vi "Init.vi"(8 "error in (no error)":errorcluster, 11 "UI in":refnum<class "UI.lvclass">) -> (0 "error out":errorcluster, 3 "UI out":refnum<class "UI.lvclass">)   [LabVIEW 2020, in "UI.lvlib" / "UI.lvclass"]
uses:
  UI.lvclass
  UI.lvclass/UI.ctl
  Read Device.vi
  Read VISA resource name.vi
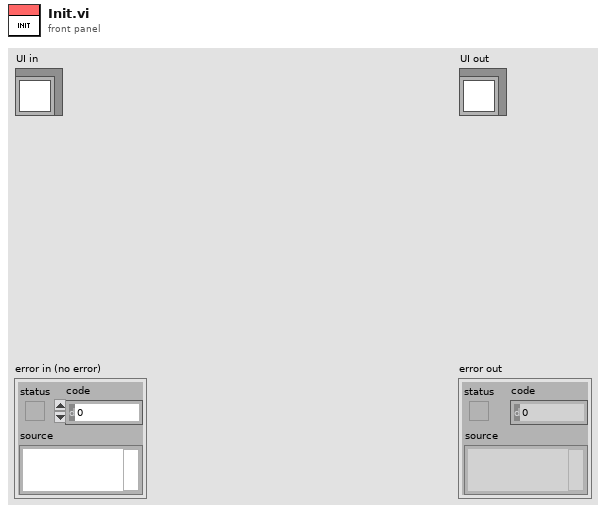
[diagram p1: front panel]
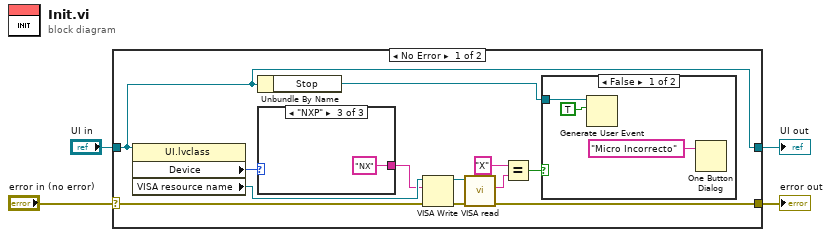
[diagram p0: block diagram]
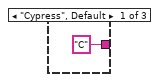
[diagram p3: hidden frame]
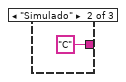
[diagram p4: hidden frame]
diagram:
  n1 = case shown="No Error" "error in (no error)" {
    selector: "error in (no error)" -> [w14 w24]
    tunnel: [w11 w24] -> w3
    tunnel: [w7 w23] -> w1
    tunnel: "UI in" -> [w7 w23]
    frame No Error {
      n2 = property class="UI.lvclass"(reference=w7) -> ("Device"=w16:enum16{"Cypress", "Simulado", "NXP"}, "VISA resource name"=w15:refnum<visa-resource-name>)  [unwired: 1 in, 2 out]
      n3 = Unbundle By Name(w7) -> ("Stop"=w6:refnum<user-event>)
      n4 = case shown="\"NXP\"" w16 {
        tunnel: ["C" "C" "NX"] -> w9
        frame "Cypress", Default {
        }
        frame "Simulado" {
        }
        frame "NXP" {
        }
      }
      n5 = VISA Write(VISA resource name=w15, write buffer=w9, error in (no error)=w14) -> (VISA resource name out=w13:refnum<visa-resource-name>, error out=w12:errorcluster)  [unwired: 1 out]
      n6 = call "VISA read.vi"("error in (no error)"=w12, "VISA Refnum in"=w13) -> ("error out"=w11:errorcluster, "String 2"=w10:string)  [unwired: 7 in, 1 out]
      n7 = Equal?(x="X", y=w10) -> (x = y?=w8:bool)
      n8 = case shown="False" w8 {
        tunnel: w6 -> [w18 _]
        frame False {
          n9 = Generate User Event(user event=w18, event data cluster=TRUE ("event data")) -> ()  [unwired: 2 in, 2 out]
          n10 = One Button Dialog(message="Micro Incorrecto") -> ()  [unwired: 1 in, 1 out]
        }
        frame True {
        }
      }
    }
    frame Error {
    }
  }
  "error out" <- w3
  "UI out" <- w1
